vi "http.post.vi"(6 "specific headers in":cluster{"header":string, "Value":string}[](array[cluster]), 7 "Content Type":string="application/json", 8 "error in":errorcluster, 9 "Request body":string, 10 "Path":string, 11 "Nominal Client in":refnum<class "Nominal Client.lvclass">) -> (0 "error out":errorcluster, 2 "Response":string, 3 "Nominal Client out":refnum<class "Nominal Client.lvclass">)   [LabVIEW 2020, in "Nominal Client.lvclass"]
uses:
  Nominal Client.lvclass
  Nominal Client.lvclass/Nominal Client.ctl
  <vilib>/JDP Science/JSONtext/LVClass Serializer/JSONtext LVClass Serializer.lvclass
  submodules/reqwest-labview/lv-src/reqwest/reqwest.lvclass
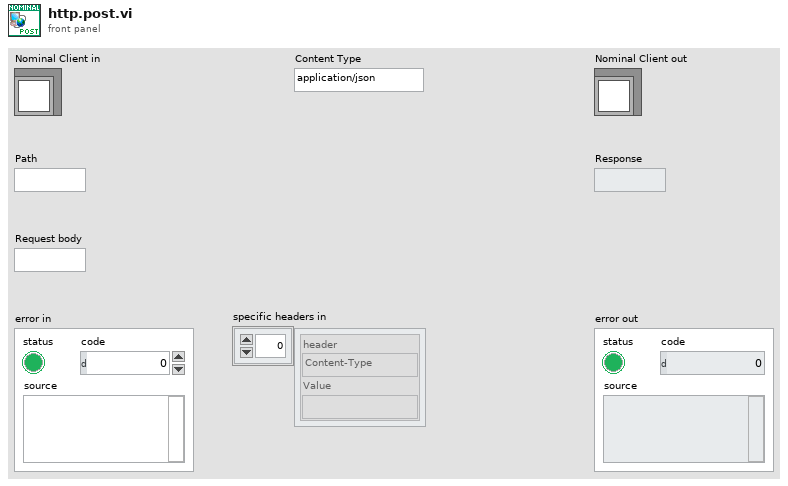
[diagram p1: front panel]
types:
  T1 = typedef "Nominal Client.lvclass/private_data.ctl" = cluster{"API Token":string, "workspace":refnum<class "workspace.lvclass">, "Available Workspaces":refnum<class "workspace.lvclass">[], "reqwest":refnum<class "reqwest.lvclass">, "timeout ms":i32}
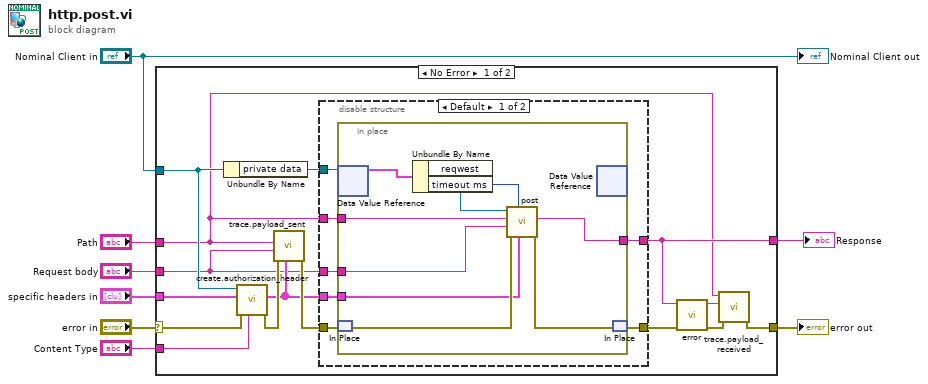
[diagram p0: block diagram]
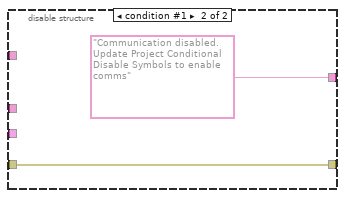
[diagram p2: hidden frame]
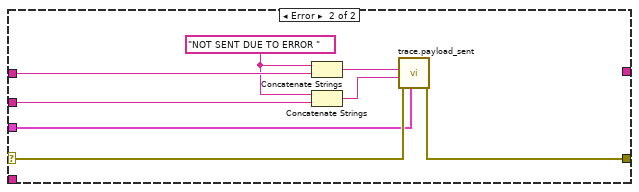
[diagram p3: hidden frame]
diagram:
  n1 = case shown="No Error" "error in" {
    selector: "error in" -> [w17 w44]
    tunnel: "Nominal Client in" -> [w21 _]
    tunnel: "specific headers in" -> [w18 w42]
    tunnel: "Request body" -> [w16 w46]
    tunnel: "Content Type" -> [w15 _]
    tunnel: [w14 _] -> w3
    tunnel: [w9 w43] -> w2
    tunnel: "Path" -> [w11 w48]
    frame No Error {
      n2 = Unbundle By Name(w21) -> ("private data"=w19:refnum<data-value>)
      n3 = call "create.authorization_header.vi"("Content Type"=w15, "error in"=w17, "specific headers in"=w18, "Nominal Client in"=w21) -> ("error out"=w23:errorcluster, "specific headers out"=w20:cluster{"header":string, "value":string}[])  [unwired: 5 in, 1 out]
      n4 = call "trace.payload_sent.vi"("Headers"=w20, "dataflow error in"=w23, "Request Body"=w16, "Path"=w11) -> ("dataflow error out"=w22:errorcluster)  [unwired: 7 in]
      n5 = disable-structure shown="Default" {
        disable-tunnel: w20 -> [w30 _]
        disable-tunnel: w19 -> [w29 _]
        disable-tunnel: w22 -> [w28 w41]
        disable-tunnel: w16 -> [w27 _]
        disable-tunnel: [w26 "Communication disabled. Update Project Conditional Disable Symbols to enable comms" ("REST Response")] -> w14
        disable-tunnel: [w25 w41] -> w12
        disable-tunnel: w11 -> [w24 _]
        frame condition #0 (active) {
          n6 = in-place {
            in-place-border: w30 -> [w35]
            in-place-border: [w37] -> w26
            in-place-border: w24 -> [w34]
            in-place-border: w27 -> [w36]
            n7 = in-place-dvr #1(w29) -> (w39:T1)  [unwired: 1 out]
            n8 = in-place-match #2(w28) -> (w38:errorcluster)
            n9 = Unbundle By Name(w39) -> ("reqwest"=w32:refnum<class "reqwest.lvclass">, "timeout ms"=w31:i32)
            n10 = call "post.vi"("request specific headers"=w35, "timeout (ms)"=w31, "error in (no error)"=w38, "request body"=w36, "path"=w34, "reqwest in"=w32) -> ("error out"=w33:errorcluster, "response"=w37:string)  [unwired: 3 in, 1 out]
            n11 = in-place-dvr #1() -> ()  [unwired: 1 in, 2 out]
            n12 = in-place-match #2(w33) -> (w25:errorcluster)
          }
        }
        frame condition #1 {
        }
      }
      n13 = call "error.vi"("error in"=w12, "REST Response"=w14) -> ("error out"=w10:errorcluster, "Error Formatted Response"=w13:string)  [unwired: 8 in]
      n14 = call "trace.payload_received.vi"("dataflow error in"=w10, "Response"=w13, "Path"=w11) -> ("dataflow error out"=w9:errorcluster)  [unwired: 8 in]
    }
    frame Error {
      w47 = "NOT SENT DUE TO ERROR " ("string")
      n15 = Concatenate Strings(w47, w48) -> (w49:string)
      n16 = Concatenate Strings(w47, w46) -> (w45:string)
      n17 = call "trace.payload_sent.vi"("Headers"=w42, "dataflow error in"=w44, "Request Body"=w45, "Path"=w49) -> ("dataflow error out"=w43:errorcluster)  [unwired: 7 in]
    }
  }
  "error out" <- w2
  "Response" <- w3
  "Nominal Client out" <- "Nominal Client in"
